vi "controlmonocromador.vi"(8 "inicio":bool, 10 "fin":dbl, 11 "inicio":dbl) -> (2 "Longitud actual":dbl)   [LabVIEW 2016]
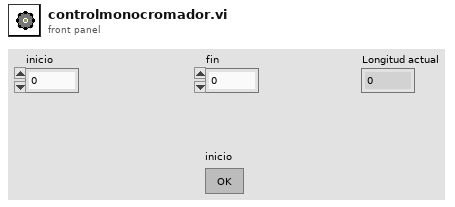
[diagram p1: front panel]
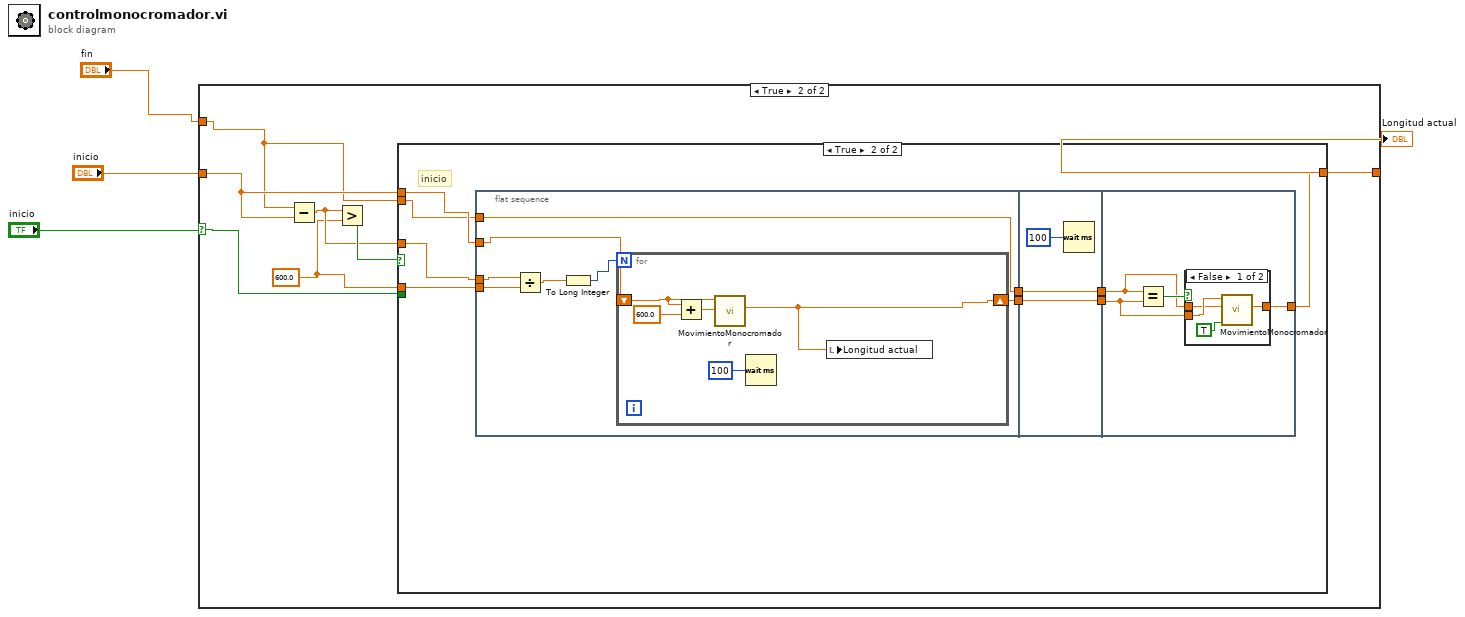
[diagram p0: block diagram]
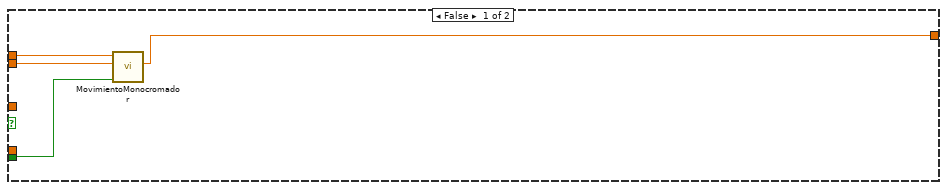
[diagram p3: hidden frame]
diagram:
  n1 = case shown="True" "inicio" {
    selector: "inicio" -> [_ w9]
    tunnel: "fin" -> [_ w10]
    tunnel: "inicio" -> [w5 w11]
    tunnel: [w5 w8] -> w1
    frame False {
    }
    frame True {
      w6 = 600.0 ("y")
      n2 = Subtract(x=w10, y=w11) -> (x-y=w7:dbl)
      n3 = Greater?(x=w7, y=w6) -> (0:w12:bool)
      n4 = case shown="True" w12 {
        tunnel: w11 -> [w16 w25]
        tunnel: w10 -> [w15 w20]
        tunnel: w9 -> [w14 _]
        tunnel: [w13 w17] -> w8
        tunnel: w7 -> [_ w24]
        tunnel: w6 -> [_ w23]
        frame False {
          n5 = call "MovimientoMonocromador.vi"("comenzar"=w14, "destino"=w15, "actual"=w16) -> ("longitud actual"=w13:dbl)  [unwired: 8 in]
        }
        frame True {
          # "inicio"
          n6 = flat-sequence {
            tunnel: w25 -> [w28]
            tunnel: w24 -> [w32]
            tunnel: w23 -> [w31]
            tunnel: [w27] -> w22
            tunnel: w20 -> [w26]
            tunnel: [w26] -> w19
            tunnel: w22 -> [w40]
            tunnel: [w40] -> w21
            tunnel: w19 -> [w38]
            tunnel: [w38] -> w18
            tunnel: w21 -> [w42]
            tunnel: w18 -> [w41]
            tunnel: [w44] -> w17
            frame #0 {
              n7 = Divide(x=w32, y=w31) -> (x/y=w30:dbl)
              n8 = To Long Integer(number=w30) -> (32bit integer=w29:i32)
              n9 = for {
                N: w29 -> [_]
                shift-right: [w34] -> w27
                shift-left: w28 -> [w36]
                n10 = Add(x=w36, y=600.0) -> (x+y=w37:dbl)
                n11 = call "MovimientoMonocromador.vi"("destino"=w37, "actual"=w36) -> ("longitud actual"=w34:dbl)  [unwired: 9 in]
                n12 = Wait (ms)(milliseconds to wait=u32 100) -> ()  [unwired: 1 out]
                n13 = local write "Longitud actual"(w34) -> ()
              }
            }
            frame #1 {
              n14 = Wait (ms)(milliseconds to wait=u32 100) -> ()  [unwired: 1 out]
            }
            frame #2 {
              n15 = Equal?(x=w41, y=w42) -> (x = y?=w43:bool)
              n16 = case shown="False" w43 {
                tunnel: [w46 w49] -> w44
                tunnel: w42 -> [w48 w49]
                tunnel: w41 -> [w47 _]
                frame False {
                  n17 = call "MovimientoMonocromador.vi"("comenzar"=TRUE, "destino"=w47, "actual"=w48) -> ("longitud actual"=w46:dbl)  [unwired: 8 in]
                }
                frame True {
                }
              }
            }
          }
        }
      }
    }
  }
  "Longitud actual" <- w1
